vi "Write Hardware Configuration.vi"(8 "error in (no error)":errorcluster, 10 "Hardware Configuration":T1={"Shutters"=[], "Stage Configuration"={"Serial Port"="COM3", "Forward Step (mm)"=0.4, "Lane Length (mm)"=6.0, "Lane Separation (mm)"=0.8, "Stage Type"=enum."Disabled"}, "Microscope Configuration"={"Serial Port"="COM2", "Microscope Type"=enum."TE2000", "FilterBlockCassette1"=refnum, "LightPathDrive"=refnum, "INikonTI"=refnum}, "Virtual Camera Configuration"={"Camera Type"=enum."Orca-Flash 4.0 V2", "Active Cameras"=[], "Sync Line"=""}, "Laser Configuration"=[], "Fluidics Configuration"={"Fluidics present"=FALSE}, "Installed Cameras"=[]}, 11 "Main Window in":refnum<class "Main Window.lvclass">) -> (0 "error out":errorcluster, 3 "Main Window out":refnum<class "Main Window.lvclass">)   [LabVIEW 2018, in "Main Window.lvlib" / "Main Window.lvclass"]
uses:
  Main Window.lvclass
  Resources/Type Defs/Hardware Configuration.ctl
  Resources/Type Defs/Shutter Configuration.ctl
  Resources/Type Defs/Stage Configuration.ctl
  Resources/Type Defs/Microscope Configuration.ctl
  Resources/Type Defs/Microscope Type.ctl
  Resources/Type Defs/Virtual Camera Configuration.ctl
  Resources/Type Defs/Camera Type.ctl
  Resources/Type Defs/Physical Camera Assignment.ctl
  Resources/Type Defs/Laser Configuration.ctl
  Resources/Type Defs/Pump Configuration.ctl
  Main Window.lvclass/Main Window.ctl
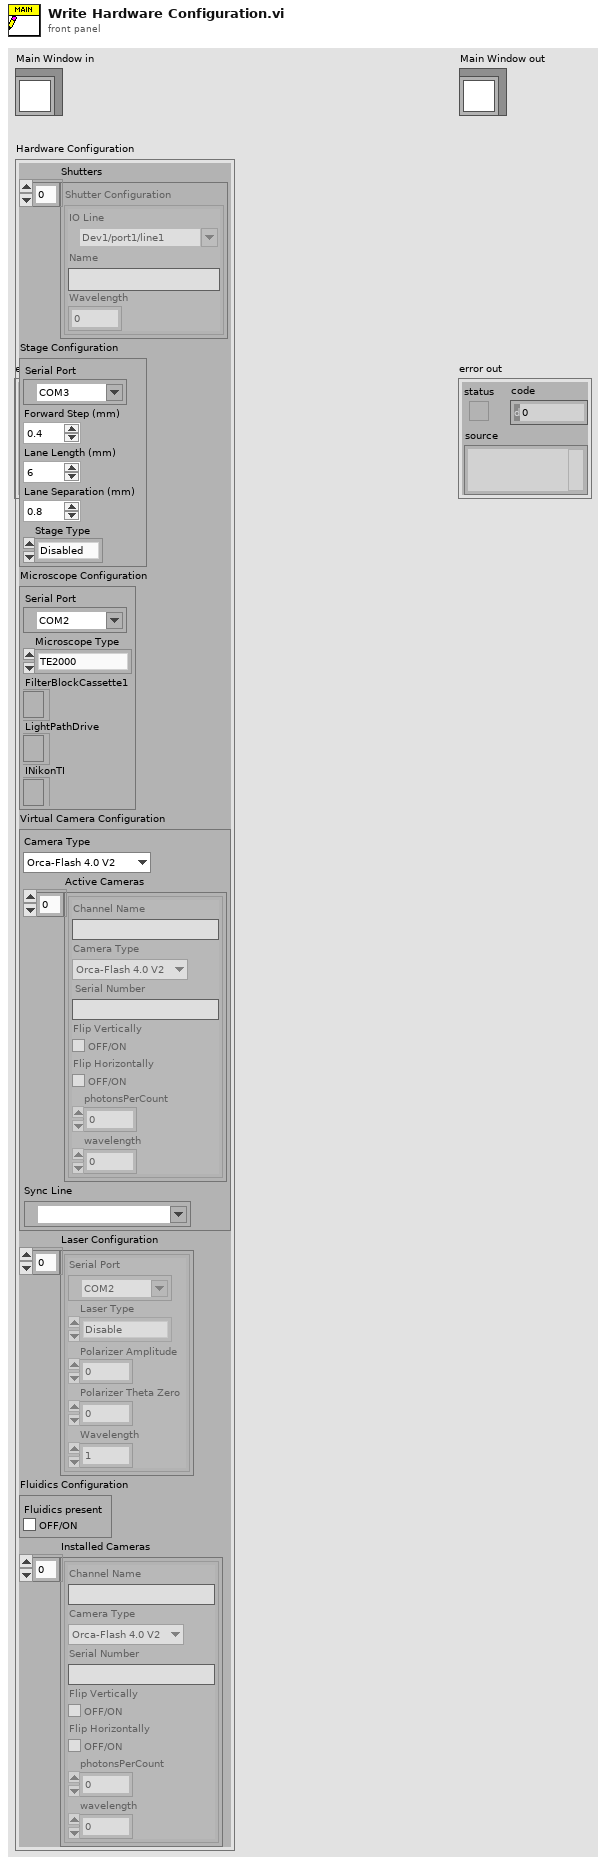
[diagram p1: front panel]
types:
  T1 = typedef "Hardware Configuration.ctl" = cluster{"Shutters":T2[], "Stage Configuration":T3, "Microscope Configuration":T4, "Virtual Camera Configuration":T6, "Laser Configuration":T9[], "Fluidics Configuration":T10, "Installed Cameras":T8[]}
  T2 = typedef "Shutter Configuration.ctl" = cluster{"IO Line":tag, "Name":string, "Wavelength":u16}
  T3 = typedef "Stage Configuration.ctl" = cluster{"Serial Port":refnum<visa-resource-name>, "Forward Step (mm)":dbl, "Lane Length (mm)":dbl, "Lane Separation (mm)":dbl, "Stage Type":enum16{"Disabled", "ESP301", "Ti2"}}
  T4 = typedef "Microscope Configuration.ctl" = cluster{"Serial Port":refnum<visa-resource-name>, "Microscope Type":T5, "FilterBlockCassette1":refnum<k7>, "LightPathDrive":refnum<k7>, "INikonTI":refnum<k7>}
  T5 = typedef "Microscope Type.ctl" = enum16{"Disable", "TE2000", "Eclipse Ti", "Ti2"}
  T6 = typedef "Virtual Camera Configuration.ctl" = cluster{"Camera Type":T7, "Active Cameras":T8[], "Sync Line":tag}
  T7 = typedef "Camera Type.ctl" = enum16{"Orca-Flash 4.0 V2"}
  T8 = typedef "Physical Camera Assignment.ctl" = cluster{"Channel Name":string, "Camera Type":T7, "Serial Number":string, "Flip Vertically":bool, "Flip Horizontally":bool, "photonsPerCount":dbl, "wavelength":i16}
  T9 = typedef "Laser Configuration.ctl" = cluster{"Serial Port":refnum<visa-resource-name>, "Laser Type":enum16{"Disable", "Laser Quantum", "Coherent OBIS", "PRM1-Z8"}, "Polarizer Amplitude":dbl, "Polarizer Theta Zero":dbl, "Wavelength":u16}
  T10 = typedef "Pump Configuration.ctl" = cluster{"Fluidics present":bool}
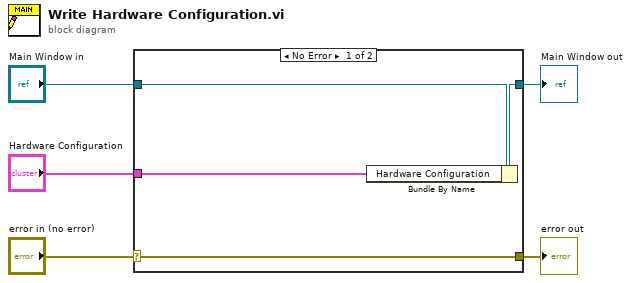
[diagram p0: block diagram]
diagram:
  n1 = case shown="No Error" "error in (no error)" {
    selector: "error in (no error)" -> [w9 w10]
    tunnel: [w9 w10] -> w4
    tunnel: [w7 w11] -> w2
    tunnel: "Main Window in" -> [w8 w11]
    tunnel: "Hardware Configuration" -> [w6 _]
    frame No Error {
      n2 = Bundle By Name(cluster=w8, "Hardware Configuration"=w6) -> (w7:refnum<class "Main Window.lvclass">)
    }
    frame Error {
    }
  }
  "error out" <- w4
  "Main Window out" <- w2
